vi "Add_Elevator_Positioning_Job.vi"(7 "New Job":bool=TRUE, 8 "error in (no error)":errorcluster, 9 "Item Edit":string, 10 "ElevatorPositionConfiguration":T1, 11 "TreeControl in":refnum<vi>) -> (0 "error out":errorcluster, 3 "TreeControl out":refnum<vi>)   [LabVIEW 2021]
uses:
  TypeDefs/ElevatorPositionConfiguration.ctl
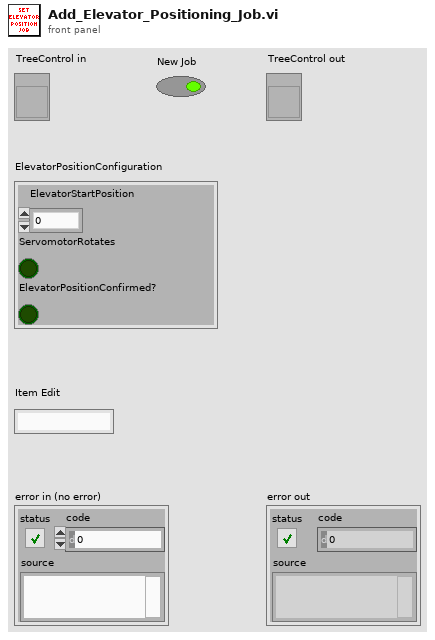
[diagram p1: front panel]
types:
  T1 = typedef "ElevatorPositionConfiguration.ctl" = cluster{"ElevatorStartPosition":dbl, "ServomotorRotates":bool, "ElevatorPositionConfirmed?":bool}
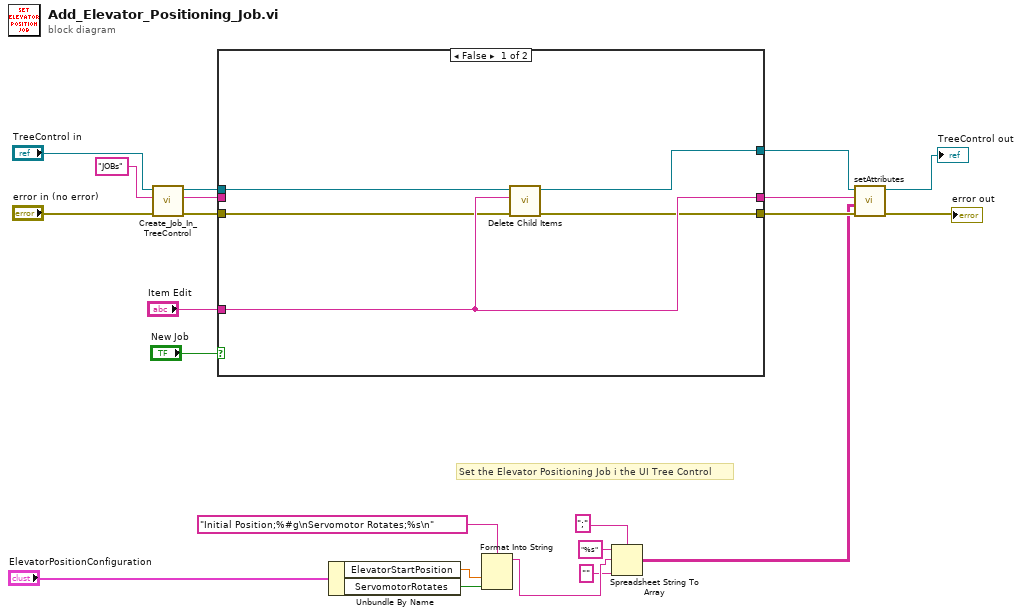
[diagram p0: block diagram]
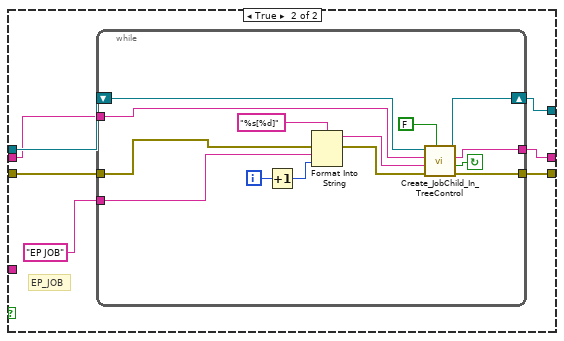
[diagram p2: hidden frame]
diagram:
  # "Set the Elevator Positioning Job i the UI Tree Control"
  n1 = call "Create_Job_In_TreeControl.vi"("error in (no error)"="error in (no error)", "Left Cell String"="JOBs", "TreeControl in"="TreeControl in") -> ("error out"=w18:errorcluster, "Edit Tree Items:Add Item"=w21:string, "TreeControl out"=w22:refnum<vi>)  [unwired: 6 in]
  n2 = case shown="False" "New Job" {
    tunnel: w22 -> [w26 w34]
    tunnel: w21 -> [_ w33]
    tunnel: w18 -> [w24 w32]
    tunnel: [w27 w31] -> w6
    tunnel: [w23 w30] -> w5
    tunnel: [w25 w29] -> w3
    tunnel: "Item Edit" -> [w27 _]
    frame False {
      n3 = call "Delete Child Items.vi"("error in (no error)"=w24, "Item Edit"=w27, "TreeControl in"=w26) -> ("error out"=w23:errorcluster, "TreeControl out"=w25:refnum<vi>)  [unwired: 7 in]
    }
    frame True {
      # "EP_JOB"
      n4 = while {
        tunnel: w32 -> [w38]
        tunnel: "EP JOB" -> [w36]
        tunnel: w33 -> [w46]
        tunnel: [w41] -> w30
        tunnel: [w40] -> w31
        shift-right: [w39] -> w29
        shift-left: w34 -> [w45]
        i -> [w43]
        stop <- w42 continue-if-true
        n5 = Increment(x=w43) -> (x+1=w35:i32)
        n6 = Format Into String(format string="%s[%d]", error in=w38, w36, w35) -> (resulting string=w47:string, error out=w37:errorcluster)  [unwired: 1 in]
        n7 = call "Create_JobChild_In_TreeControl.vi"("Child Only?"=FALSE, "error in (no error)"=w37, "Child Tag Name"=w47, "Parent Item"=w46, "TreeControl in"=w45) -> ("error out"=w41:errorcluster, "Tag Already Exists?"=w42:bool, "Edit Tree Items:Add Item 2"=w40:string, "TreeControl out"=w39:refnum<vi>)  [unwired: 3 in]
      }
    }
  }
  n8 = Unbundle By Name("ElevatorPositionConfiguration") -> ("ElevatorStartPosition"=w15:dbl, "ServomotorRotates"=w16:bool)
  n9 = Format Into String(format string="Initial Position;%#g\nServomotor Rotates;%s\n", w15, w16) -> (resulting string=w12:string)  [unwired: 2 in, 1 out]
  n10 = Spreadsheet String To Array(delimiter (Tab)=";" ("delimiter"), format string="%s", spreadsheet string=w12, array type (2D Dbl)="" ("format string")) -> (array=w4:string[][])
  n11 = call "setAttributes.vi"("error in (no error)"=w5, "Array"=w4, "Edit Tree Items:Add Item in"=w6, "TreeControl in"=w3) -> ("error out"=→"error out":errorcluster, "TreeControl out"=→"TreeControl out":refnum<vi>)  [unwired: 6 in]
